vi "heater_control.vi"() -> ()   [LabVIEW 2016]
uses:
  <instrlib>/Phidgets/Phidget Temperature Sensor/Public/TemperatureSensorStart.vi
  <instrlib>/Phidgets/Phidget Digital Output/Public/DigitalOutputOpen.vi
  <instrlib>/Phidgets/Phidget Digital Output/Public/DigitalOutputClose.vi
  <instrlib>/Phidgets/Phidget Temperature Sensor/Public/TemperatureSensorClose.vi
  <instrlib>/Phidgets/Phidget Temperature Sensor/Phidget Temperature Sensor.lvlib
  <instrlib>/Phidgets/Phidget Common/Phidget Common.lvlib
  <instrlib>/Phidgets/Phidget Digital Output/Phidget Digital Output.lvlib
panel:
  out "Waveform Chart":dbl(graph)
  out "CO2 Temperature (C)":dbl caption="Temperature"
  in  "Heater on timing (s)":dbl=30.0 caption="Time Target (s)"
  out "Attached? 2":bool caption="Attached?"
  out "Attached?":bool
  in  "Relays":T1={"Serial Number"=257915, "Channel"=0, "Port"=0} caption="Device Info"
  in  "stop":bool
  in  "Thermocouple sample rate (MS)":i32=100 caption="Data Interval"
  in  "ThermocoupleType":u32(ring)=4 items=["THERMOCOUPLE_TYPE_J"=1, "THERMOCOUPLE_TYPE_K"=2, "THERMOCOUPLE_TYPE_E"=3, "THERMOCOUPLE_TYPE_T"=4]
  in  "Thermocouple":T1={"Serial Number"=167005, "Channel"=0, "Port"=0} caption="Device Info"
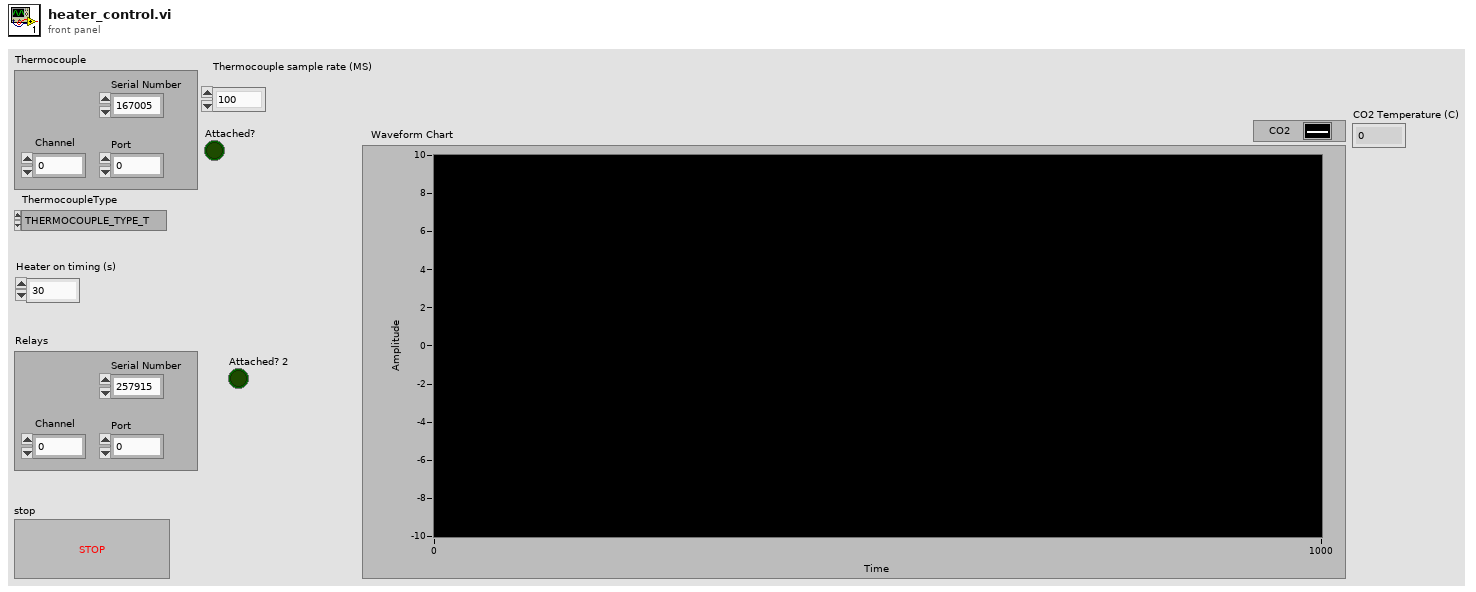
[diagram p1: front panel]
types:
  T1 = cluster{"Serial Number":i32, "Channel":i32, "Port":i32}
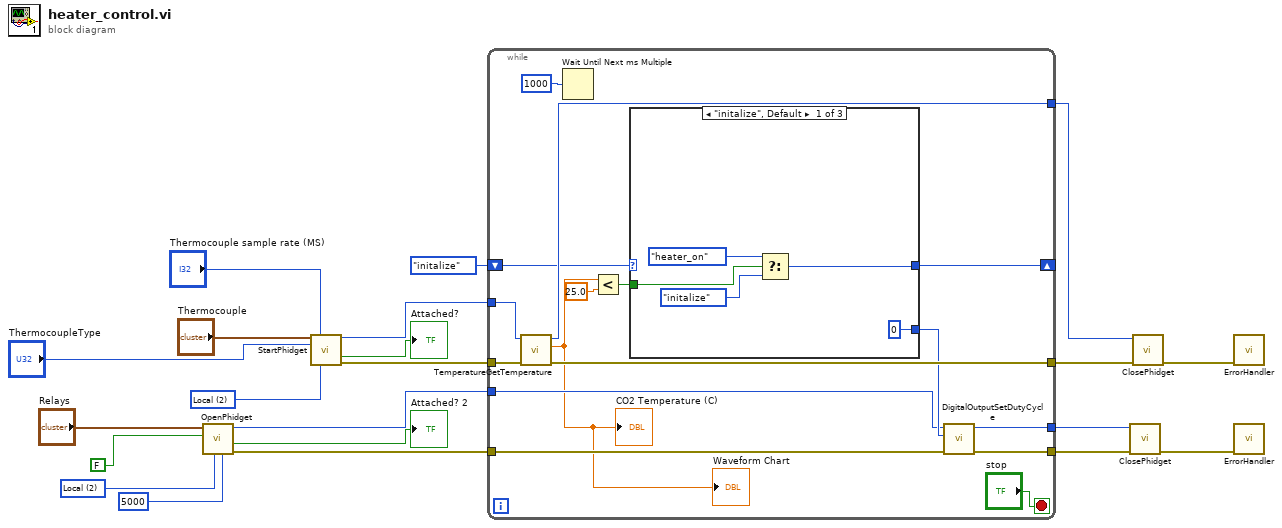
[diagram p0: block diagram]
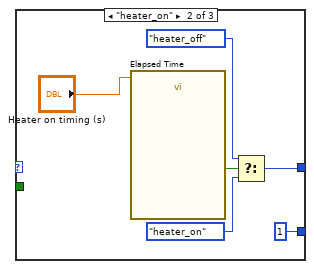
[diagram p2: hidden frame]
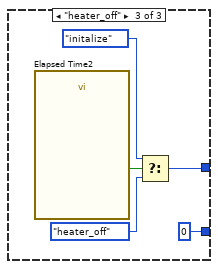
[diagram p3: hidden frame]
diagram:
  w8 = u16 2 items=["No Preference", "Remote", "Local"] ("Connection")
  w14 = u16 2 items=["No Preference", "Remote", "Local"] ("Connection")
  n1 = call-poly <instrlib>:"OpenPhidget.vi"("Timeout (mSec)"=5000, "Connection"=w8, "IsHubPort"=FALSE, "Device Info"="Relays") -> ("error out"=w4:errorcluster, "Attached?"=→"Attached? 2":bool, "Phidget ID"=w5:u64)  [unwired: 4 in, 1 out]
  n2 = call-poly <instrlib>:"StartPhidget.vi"("Device Info"="Thermocouple", "Data Interval"="Thermocouple sample rate (MS)", "ThermocoupleType"="ThermocoupleType", "Connection"=w14) -> ("Phidget ID"=w18:u64, "Attached?"=→"Attached?":bool, "error out"=w17:errorcluster)  [unwired: 8 in, 1 out]
  n3 = while {
    tunnel: w18 -> [w37]
    tunnel: w17 -> [w36]
    tunnel: [w34] -> w16
    tunnel: [w33] -> w15
    shift-right: [w28] -> _
    shift-left: enum16{"initalize", "heater_on", "heater_off"}."initalize" -> [w30]
    tunnel: w5 -> [w26]
    tunnel: w4 -> [w25]
    tunnel: [w24] -> w3
    tunnel: [w23] -> w2
    stop <- "stop" stop-if-true
    n4 = call <instrlib>:"TemperatureGetTemperature.vi"("error in (no error)"=w36, "Device In"=w37) -> ("error out"=w33:errorcluster, "temperature"=w22:dbl, "Device Out"=w34:u64)  [unwired: 6 in]
    "CO2 Temperature (C)" <- w22
    "Waveform Chart" <- w22
    n5 = Wait Until Next ms Multiple(millisecond multiple=u32 1000) -> ()  [unwired: 1 out]
    n6 = Less?(x=w22, y=25.0) -> (x < y?=w29:bool)
    n7 = case shown="\"initalize\", Default" w30 {
      tunnel: w29 -> [w42 _ _]
      tunnel: [w39 w44 w49] -> w28
      tunnel: [u8 0 ("State") u8 1 ("State") u8 0 ("State")] -> w27
      frame "initalize", Default {
        n8 = Select(t=enum16{"initalize", "heater_on", "heater_off"}."heater_on", s=w42, f=enum16{"initalize", "heater_on", "heater_off"}."initalize") -> (s? t:f=w39:enum16{"initalize", "heater_on", "heater_off"})
      }
      frame "heater_on" {
        n9 = call "Elapsed Time"("Time Target (s)"="Heater on timing (s)") -> ("Time has Elapsed"=w47:bool)  [unwired: 11 in, 7 out]
        n10 = Select(t=enum16{"initalize", "heater_on", "heater_off"}."heater_off", s=w47, f=enum16{"initalize", "heater_on", "heater_off"}."heater_on") -> (s? t:f=w44:enum16{"initalize", "heater_on", "heater_off"})
      }
      frame "heater_off" {
        n11 = call "Elapsed Time2"() -> ("Time has Elapsed"=w52:bool)  [unwired: 12 in, 7 out]
        n12 = Select(t=enum16{"initalize", "heater_on", "heater_off"}."initalize", s=w52, f=enum16{"initalize", "heater_on", "heater_off"}."heater_off") -> (s? t:f=w49:enum16{"initalize", "heater_on", "heater_off"})
      }
    }
    n13 = call <instrlib>:"DigitalOutputSetDutyCycle.vi"("error in (no error)"=w25, "Duty Cycle"=w27, "Device In"=w26) -> ("error out"=w23:errorcluster, "Device Out"=w24:u64)  [unwired: 6 in]
  }
  n14 = call-poly <instrlib>:"ClosePhidget.vi"("error in"=w2, "Device In"=w3) -> ("error out"=w1:errorcluster)  [unwired: 9 in]
  n15 = call-poly <instrlib>:"ClosePhidget.vi"("error in"=w15, "Device In"=w16) -> ("error out"=w9:errorcluster)  [unwired: 9 in]
  n16 = call <instrlib>:"ErrorHandler.vi"("error in"=w9) -> ()  [unwired: 9 in, 2 out]
  n17 = call <instrlib>:"ErrorHandler.vi"("error in"=w1) -> ()  [unwired: 9 in, 2 out]
